vi "Time_series_exam.vi"(8 "error in":errorcluster, 9 "Plot reference":refnum<vi>, 10 "Abort":refnum<vi>, 11 "Centre VI":refnum<vi>) -> (0 "error out":errorcluster)   [LabVIEW 2016]
panel:
  in  "Autoscale Y":bool=TRUE
  in  "Autoscale X":bool=TRUE
  in  "Cancel":bool
  in  "OK":bool
  in  "Stop":bool
  out "Time series trace":cluster{"Time":dbl[], "Data":dbl[]}[](graph) caption="XY Graph"
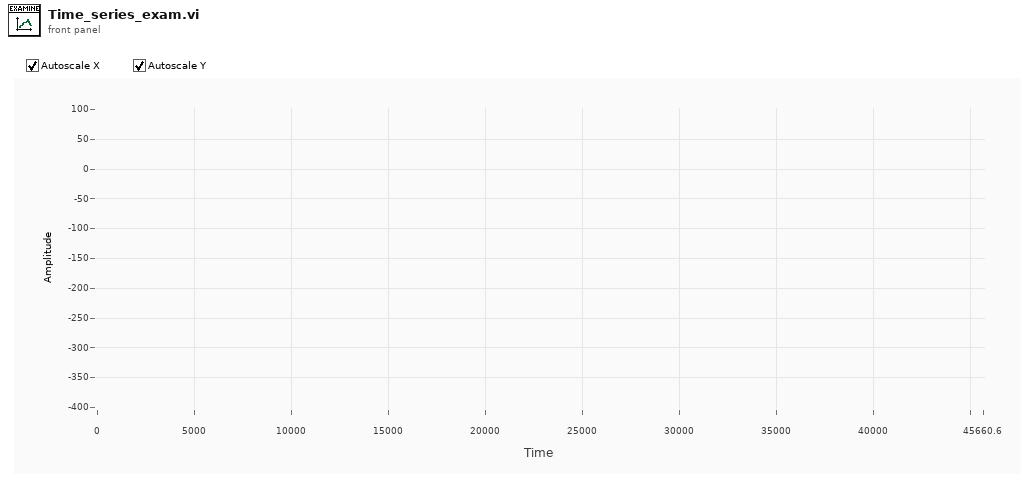
[diagram p1: front panel]
types:
  T1 = enum32{"Invalid", "Standard", "Closed", "Hidden", "Minimized", "Maximized"}
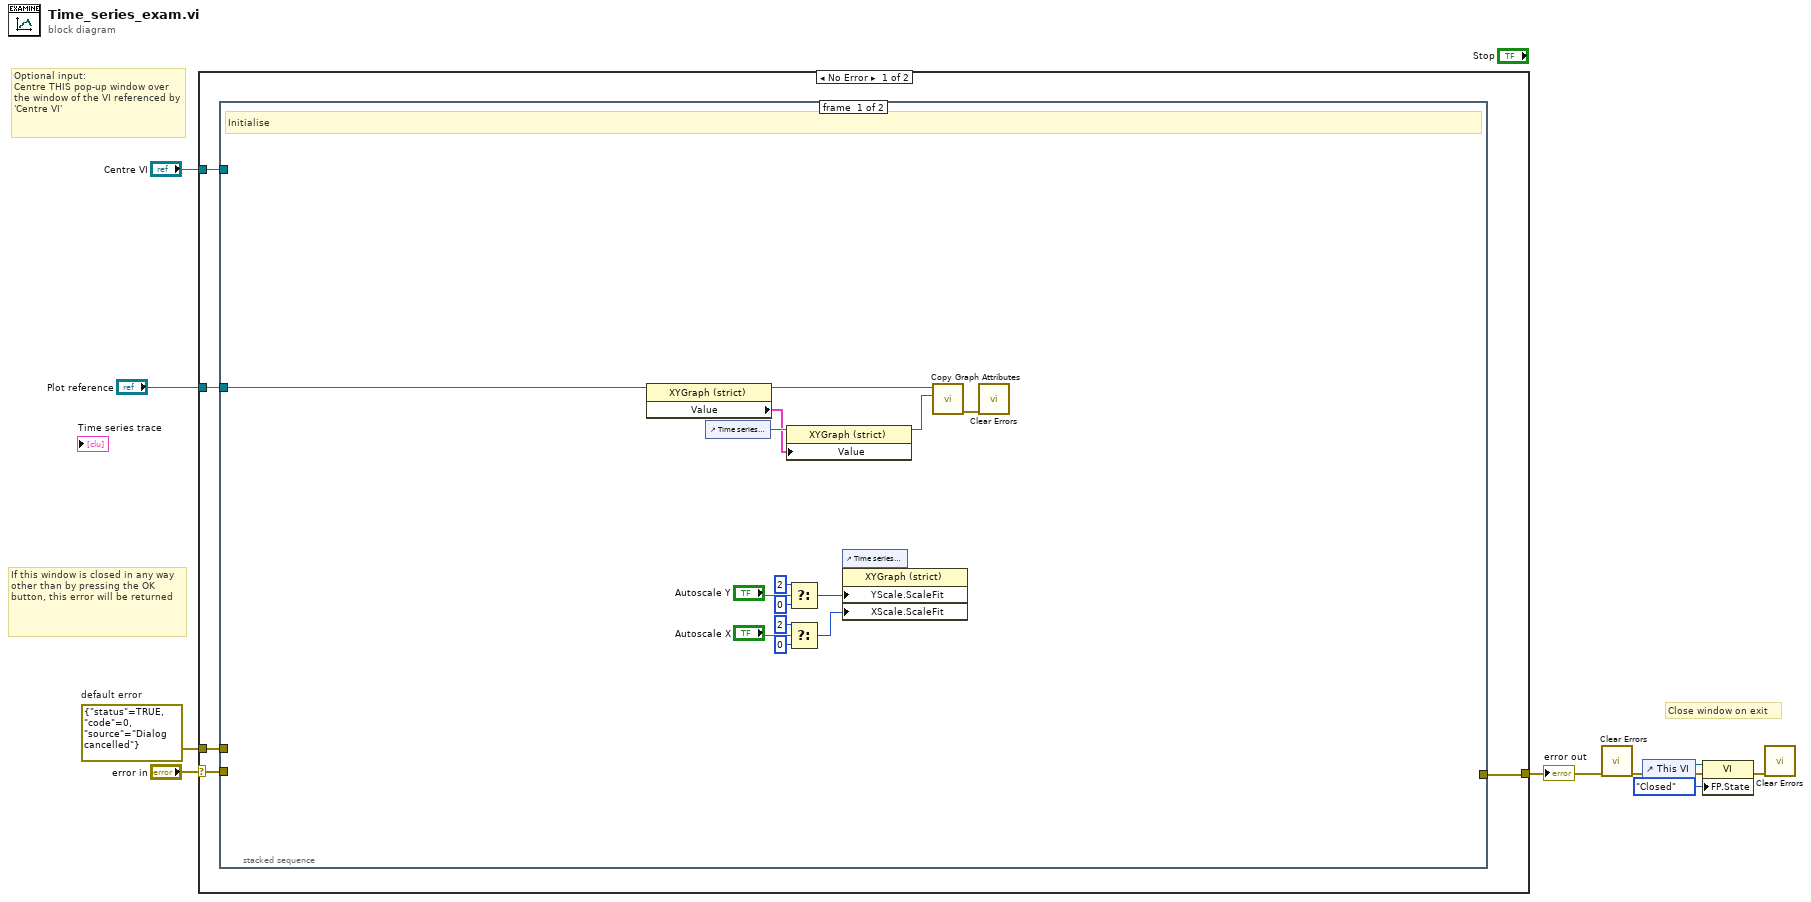
[diagram p0: block diagram]
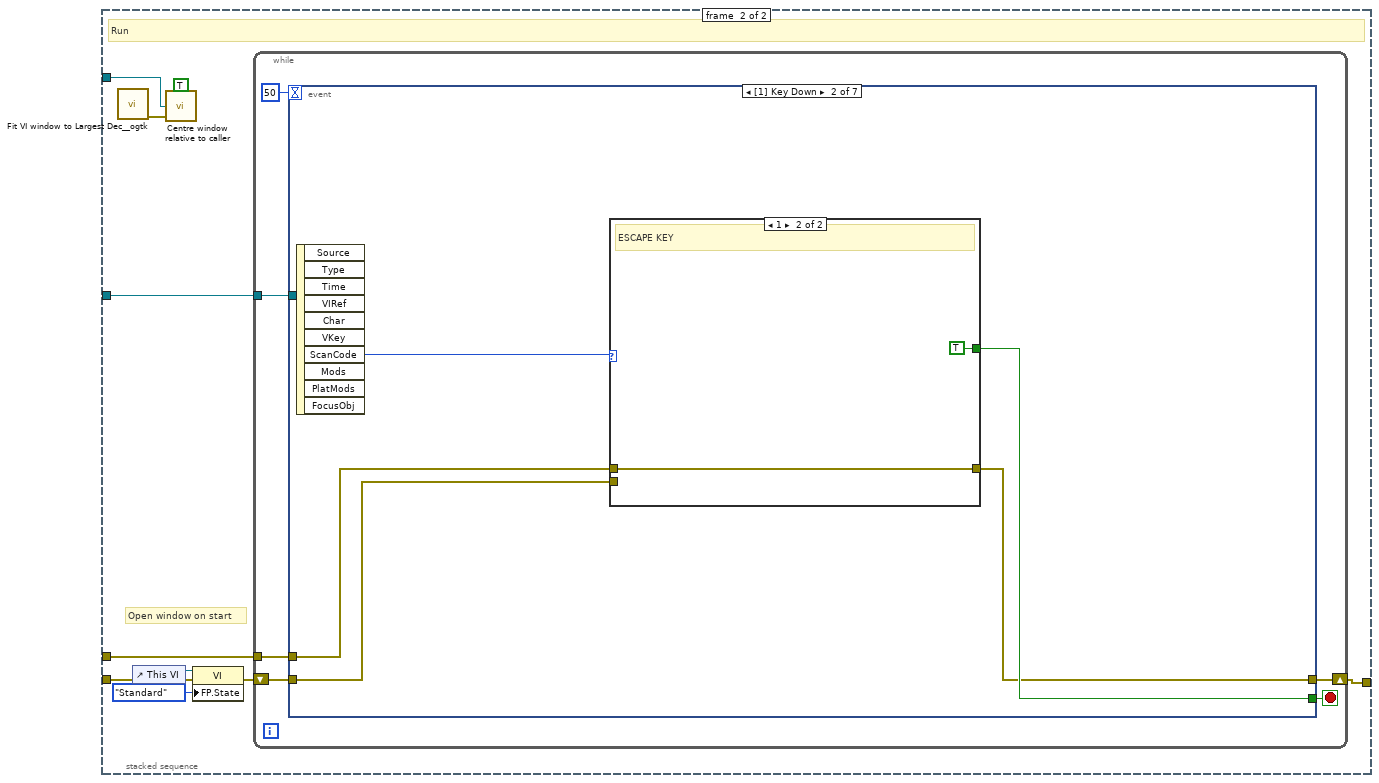
[diagram p2: hidden frame]
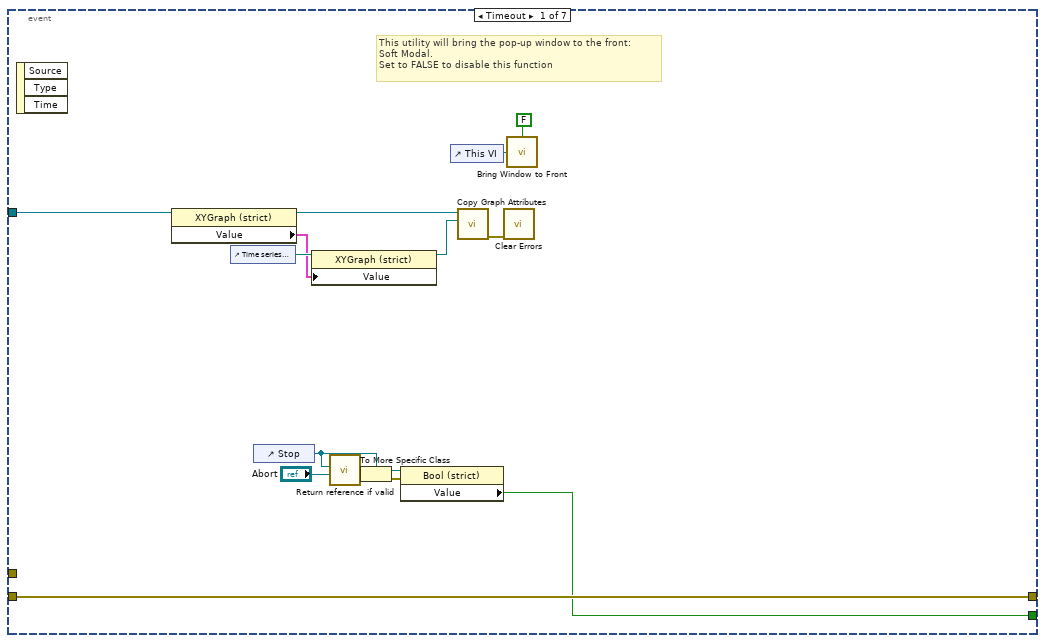
[diagram p3: hidden frame]
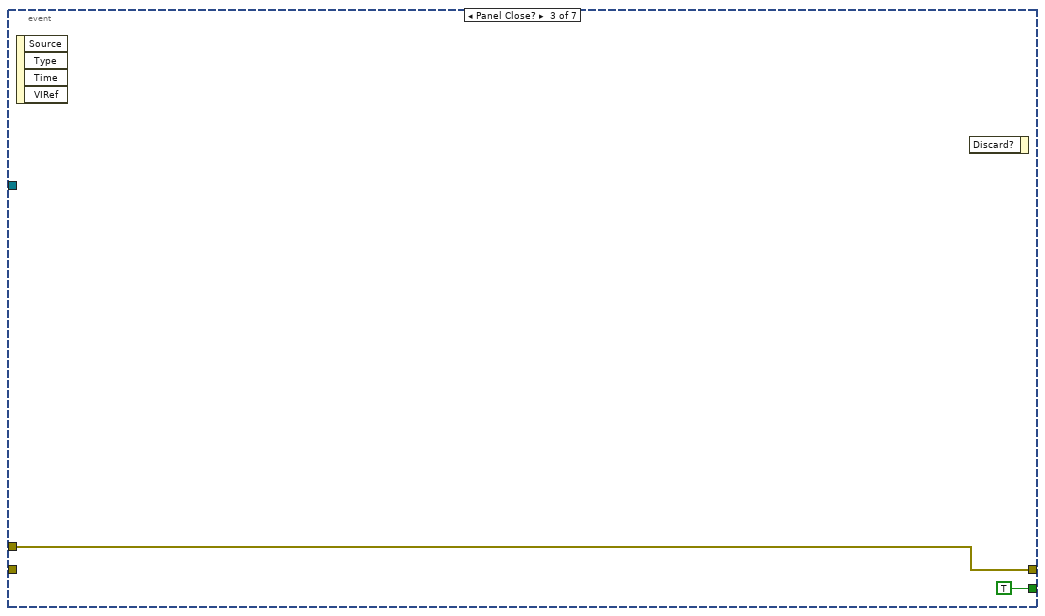
[diagram p5: hidden frame]
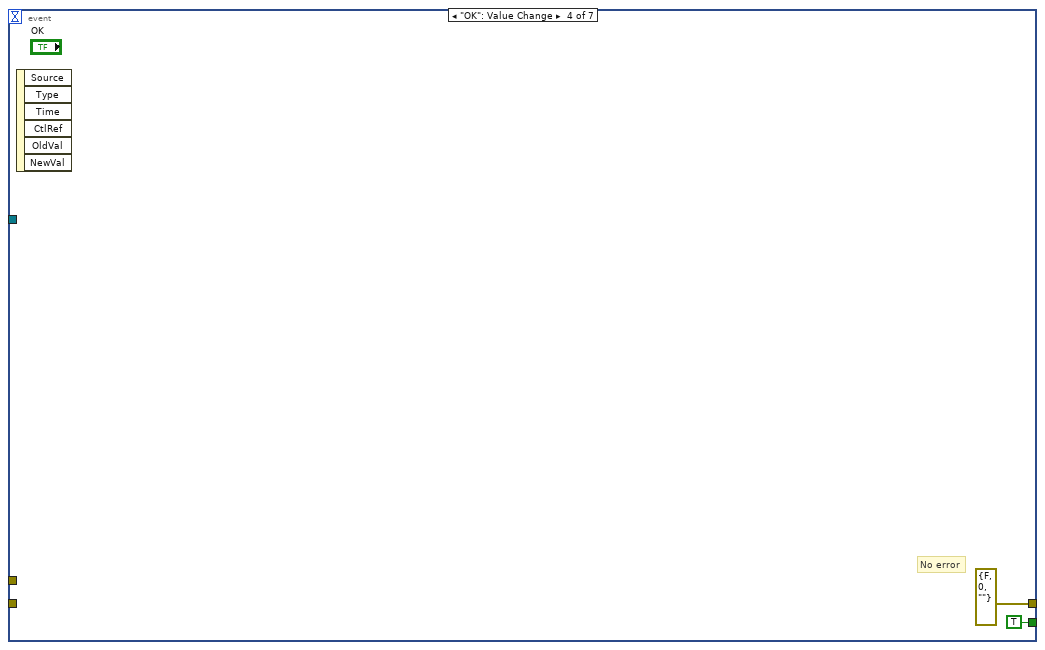
[diagram p6: hidden frame]
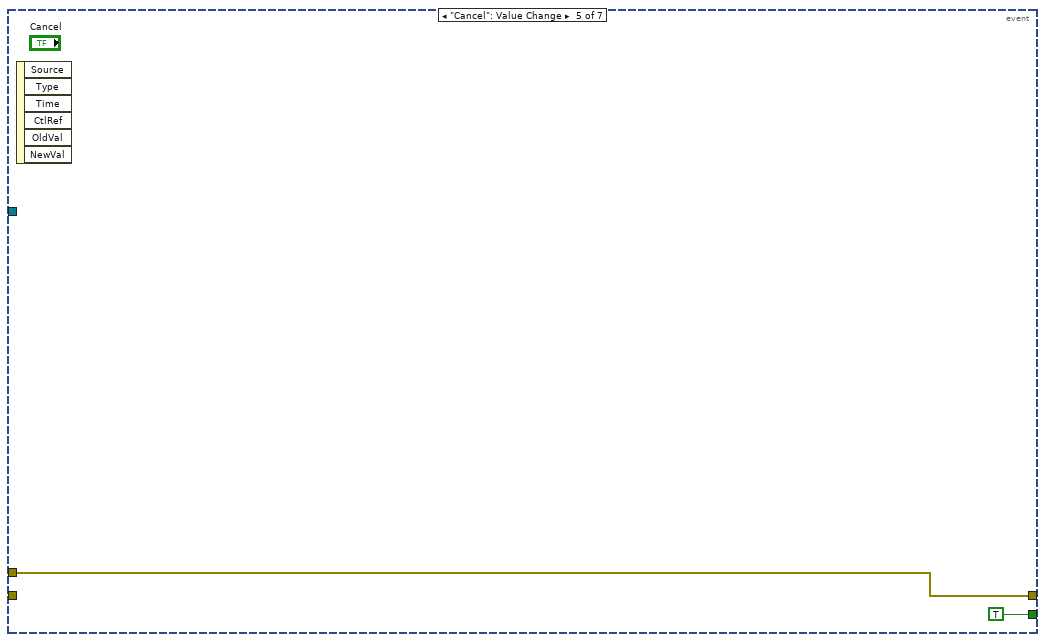
[diagram p7: hidden frame]
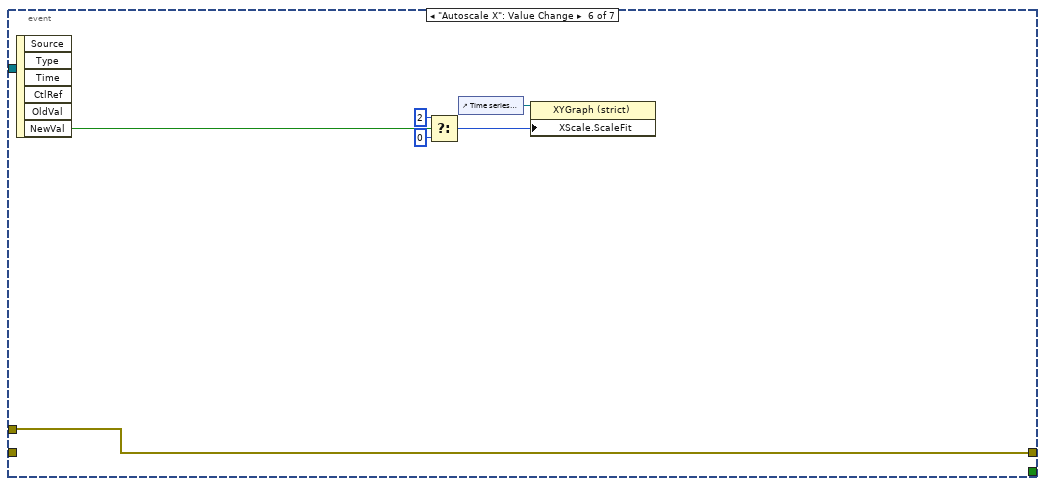
[diagram p8: hidden frame]
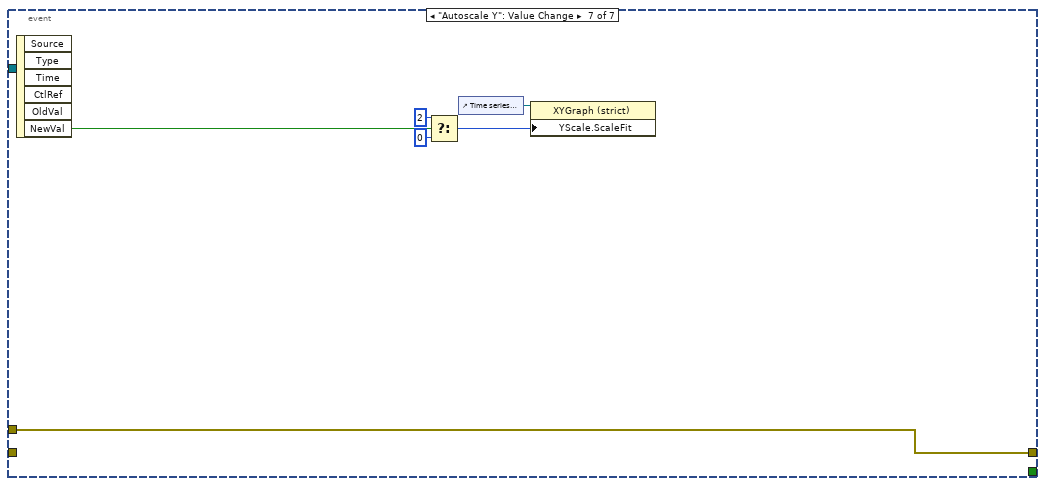
[diagram p9: hidden frame]
diagram:
  w3 = errorcluster {"status"=TRUE, "code"=0, "source"="Dialog cancelled"}  # default error
  # "Close window on exit"
  # "If this window is closed in any way other than by pressing the OK button, this error will be returned"
  # "Optional input:\nCentre THIS pop-up window over the window of the VI referenced by 'Centre VI'"
  n1 = case shown="No Error" "error in" {
    selector: "error in" -> [w11 w87]
    tunnel: [w14 w87] -> w8
    tunnel: w3 -> [w12 _]
    tunnel: "Centre VI" -> [w13 _]
    tunnel: "Plot reference" -> [w10 _]
    frame No Error {
      n2 = stacked-sequence {
        tunnel: w11 -> [_ w38]
        tunnel: [_ w39] -> w14
        tunnel: w13 -> [_ w32]
        tunnel: w12 -> [_ w31]
        tunnel: w10 -> [w15 w30]
        frame #0 {
          # "Initialise"
          n3 = property class="XYGraph (strict)"(reference=w15) -> (reference out=w17:refnum<vi>, "Value"=w16:cluster{"Time":dbl[], "Data":dbl[]}[])  [unwired: 1 in, 1 out]
          n4 = control-ref of="Time series trace"() -> (w19:refnum<vi>)
          n5 = property class="XYGraph (strict)"(reference=w19, "Value"=w16) -> (reference out=w18:refnum<vi>)  [unwired: 1 in, 1 out]
          n6 = Select(t=u8 2 ("f"), s="Autoscale Y", f=u8 0) -> (s? t:f=w25:u8)
          n7 = Select(t=u8 2 ("f"), s="Autoscale X", f=u8 0) -> (s? t:f=w21:u8)
          n8 = control-ref of="Time series trace"() -> (w29:refnum<vi>)
          n9 = property class="XYGraph (strict)"(reference=w29, "YScale.ScaleFit"=w25, "XScale.ScaleFit"=w21) -> ()  [unwired: 1 in, 2 out]
          n10 = call "Copy Graph Attributes.vi"("Copy to"=w18, "Copy from"=w17) -> ("error out"=w20:errorcluster)  [unwired: 9 in]
          n11 = call <vilib>:"Clear Errors.vi"("error in (no error)"=w20) -> ()  [unwired: 5 in, 2 out]
        }
        frame #1 {
          # "Open window on start"
          # "Run"
          n12 = call <userlib>:"Fit VI window to Largest Dec__ogtk.vi"() -> ("error out"=w33:errorcluster)  [unwired: 6 in, 1 out]
          n13 = control-ref of="This VI"() -> (w35:refnum<vi>)
          n14 = call <userlib>:"Centre window relative to caller.vi"("Enable (T)"=TRUE, "error in"=w33, "VI reference"=w32) -> ()  [unwired: 2 in, 1 out]
          n15 = property class="VI"(reference=w35, error in=w38, "FP.State"=T1."Standard" ("Front Panel Window:State")) -> (error out=w37:errorcluster)  [unwired: 1 out]
          n16 = while {
            shift-right: [w43] -> w39
            shift-left: w37 -> [w42]
            tunnel: w31 -> [w41]
            tunnel: w30 -> [w40]
            stop <- w45 stop-if-true
            n17 = event shown="[1] Key Down" {
              selector: _ -> [_ _ _ _ _ _ _]
              dyn-events: _ -> [_ _ _ _ _ _ _]
              timeout: 50 -> [_ _ _ _ _ _ _]
              tunnel: [w52 w64 TRUE TRUE TRUE _ _] -> w45
              tunnel: [w59 w62 w69 errorcluster {"status"=FALSE, "code"=0, "source"=""} ("error in (no error)") w73 w75 w81] -> w43
              tunnel: w42 -> [w59 w61 _ _ _ _ _]
              tunnel: w41 -> [_ w63 w69 _ w73 w75 w81]
              tunnel: w40 -> [w48 _ _ _ _ _ _]
              event Timeout {
                # "This utility will bring the pop-up window to the front:\nSoft Modal.\nSet to FALSE to disable this function"
                n18 = event-data() -> ()  [unwired: 1 in, 3 out]
                n19 = property class="XYGraph (strict)"(reference=w48) -> (reference out=w47:refnum<vi>, "Value"=w46:cluster{"Time":dbl[], "Data":dbl[]}[])  [unwired: 1 in, 1 out]
                n20 = control-ref of="Time series trace"() -> (w50:refnum<vi>)
                n21 = control-ref of="Stop"() -> (w53:refnum<vi>)
                n22 = property class="XYGraph (strict)"(reference=w50, "Value"=w46) -> (reference out=w49:refnum<vi>)  [unwired: 1 in, 1 out]
                n23 = call <userlib>:"Return reference if valid.vi"("Default"=w53, "Preferred"="Abort") -> ("Reference"=w57:refnum<vi>)  [unwired: 5 in]
                n24 = To More Specific Class(target class=w53, reference=w57) -> (specific class reference=w55:refnum<vi>, error out=w54:errorcluster)  [unwired: 1 in]
                n25 = property on="Property Node" class="Bool (strict)"(reference=w55, error in=w54) -> ("Value"=w52:bool)  [unwired: 2 out]
                n26 = control-ref of="This VI"() -> (w58:refnum<vi>)
                n27 = call "Copy Graph Attributes.vi"("Copy to"=w49, "Copy from"=w47) -> ("error out"=w51:errorcluster)  [unwired: 9 in]
                n28 = call <vilib>:"Clear Errors.vi"("error in (no error)"=w51) -> ()  [unwired: 5 in, 2 out]
                n29 = call <userlib>:"Bring Window to Front.vi"("Enable (T)"=FALSE, "VI reference"=w58) -> ()  [unwired: 4 in]
              }
              event Key Down {
                n30 = event-data() -> ("ScanCode"=w65:i16)  [unwired: 1 in, 9 out]
                n31 = case shown="1" w65 {
                  tunnel: [_ TRUE] -> w64
                  tunnel: [w66 w67] -> w62
                  tunnel: w63 -> [_ w67]
                  tunnel: w61 -> [w66 _]
                  frame 0, Default {
                  }
                  frame 1 {
                    # "ESCAPE KEY"
                  }
                }
              }
              event Panel Close? {
                n32 = event-data() -> ()  [unwired: 1 in, 4 out]
                n33 = event-data() -> ()  [unwired: 2 in, 1 out]
              }
              event "OK": Value Change {
                # "No error"
                n34 = event-data() -> ()  [unwired: 1 in, 6 out]
              }
              event "Cancel": Value Change {
                n35 = event-data() -> ()  [unwired: 1 in, 6 out]
              }
              event "Autoscale X": Value Change {
                n36 = event-data() -> ("NewVal"=w76:bool)  [unwired: 1 in, 5 out]
                n37 = Select(t=u8 2 ("f"), s=w76, f=u8 0) -> (s? t:f=w77:u8)
                n38 = control-ref of="Time series trace"() -> (w80:refnum<vi>)
                n39 = property class="XYGraph (strict)"(reference=w80, "XScale.ScaleFit"=w77) -> ()  [unwired: 1 in, 2 out]
              }
              event "Autoscale Y": Value Change {
                n40 = event-data() -> ("NewVal"=w82:bool)  [unwired: 1 in, 5 out]
                n41 = Select(t=u8 2 ("f"), s=w82, f=u8 0) -> (s? t:f=w83:u8)
                n42 = control-ref of="Time series trace"() -> (w86:refnum<vi>)
                n43 = property class="XYGraph (strict)"(reference=w86, "YScale.ScaleFit"=w83) -> ()  [unwired: 1 in, 2 out]
              }
            }
          }
        }
      }
    }
    frame Error {
    }
  }
  "error out" <- w8
  n44 = call <vilib>:"Clear Errors.vi"("error in (no error)"=w8) -> ("error out"=w7:errorcluster)  [unwired: 5 in, 1 out]
  n45 = control-ref of="This VI"() -> (w5:refnum<vi>)
  n46 = property class="VI"(reference=w5, error in=w7, "FP.State"=T1."Closed" ("Front Panel Window:State")) -> (error out=w9:errorcluster)  [unwired: 1 out]
  n47 = call <vilib>:"Clear Errors.vi"("error in (no error)"=w9) -> ()  [unwired: 5 in, 2 out]
